vi "Get One-Port Charact Data.vi"(0 "Cal Standard in":refnum<class "Cal Standard Base.lvclass">, 5 "Port Name":string, 11 "error in (no error)":errorcluster) -> (4 "Cal Standard out":refnum<class "Cal Standard Base.lvclass">, 6 "Found":bool, 8 "One-Port Charact Data":T1[](array[typedef]), 15 "error out":errorcluster)   [LabVIEW 2023, in "RFFixtureCharact.Instruments.lvlib" / "Cal Standard Base.lvclass"]
uses:
  Cal Standard Base.lvclass
  Type Definitions/One-Port Charact Data.ctl
  Type Definitions/Standard Type.ctl
  Properties/Read One-Port Cal Standards.vi
  RFFixtureCharact.Instruments.lvlib
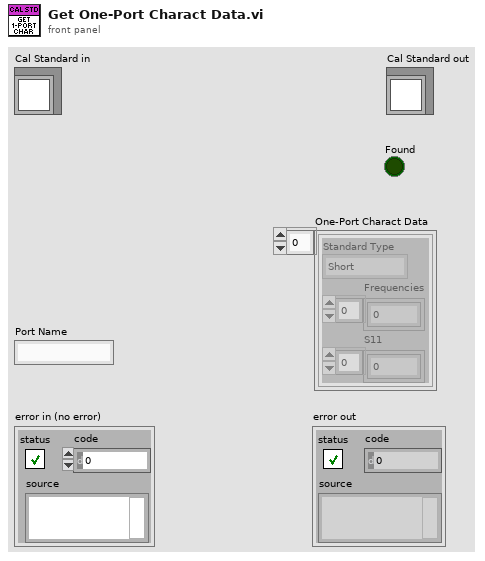
[diagram p1: front panel]
types:
  T1 = typedef "RFFixtureCharact.Instruments.lvlib/One-Port Charact Data.ctl" = cluster{"Standard Type":T2, "Frequencies":dbl[], "S11":cdb[]}
  T2 = typedef "RFFixtureCharact.Instruments.lvlib/Standard Type.ctl" = enum16{"Short", "Open", "Load"}
  T3 = typedef "RFFixtureCharact.Instruments.lvlib/One-Port Cal Standard.ctl" = cluster{"Port Name":string, "Charact Data":T1[]}
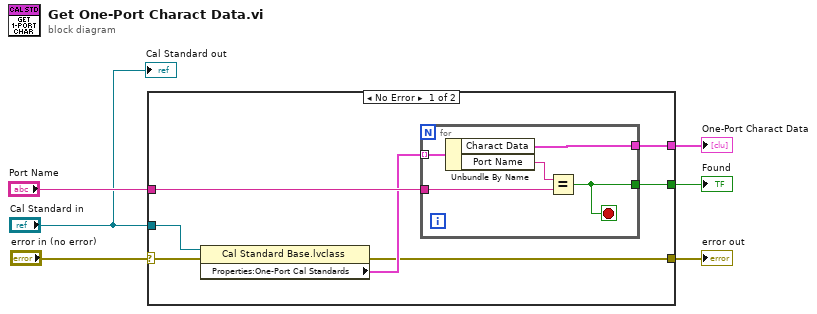
[diagram p0: block diagram]
diagram:
  n1 = case shown="No Error" "error in (no error)" {
    selector: "error in (no error)" -> [w11 w19]
    tunnel: "Port Name" -> [w13 _]
    tunnel: [w12 _] -> w5
    tunnel: [w8 w19] -> w3
    tunnel: "Cal Standard in" -> [w10 _]
    tunnel: [w7 _] -> w1
    frame No Error {
      n2 = property class="Cal Standard Base.lvclass"(reference=w10, error in=w11) -> (error out=w8:errorcluster, "Properties:One-Port Cal Standards"=w9:T3[])  [unwired: 1 out]
      n3 = for {
        tunnel: w9 -> [w18] mode=indexing
        tunnel: w13 -> [w15]
        tunnel: [w17] -> w12
        tunnel: [w14] -> w7
        stop <- w14 stop-if-true
        n4 = Unbundle By Name(w18) -> ("Charact Data"=w17:T1[], "Port Name"=w16:string)
        n5 = Equal?(x=w16, y=w15) -> (x = y?=w14:bool)
      }
    }
    frame Error {
    }
  }
  "One-Port Charact Data" <- w5
  "error out" <- w3
  "Found" <- w1
  "Cal Standard out" <- "Cal Standard in"
